vi "Load XML.vi"(8 "Error In":errorcluster, 10 "XML File":path caption="UIM XML Path", 11 "UIM In":refnum<data-value>) -> (0 "Error Out":errorcluster, 3 "UIM Out":refnum<data-value>)   [LabVIEW 2020, in "UIM.lvlib" / "UIM.lvclass"]
doc: "Overwrite the existing UIM state data with the data loaded from XML.\n\n<b>Important </b>- If the XML file specifies the <UIPList> only the plugins specified in that list will be used and loaded with the file. Make sure that the list specifies ALL the plugins used in the UIM States. Otherwise they will not be loaded. If the <UIPList> is not present in the file then the default UIPs and the UIPs from the Plugin folder will be used."
uses:
  UIM.lvclass
  <vilib>/xml/Load XML File.vi
  <vilib>/xml/Close Reference(Node).vi
  <vilib>/xml/NI_XML.lvlib
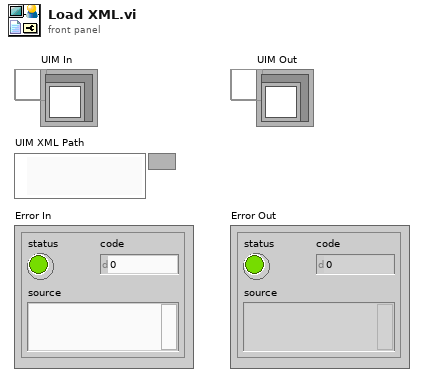
[diagram p1: front panel]
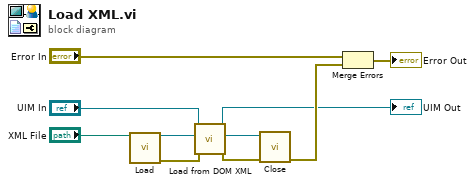
[diagram p0: block diagram]
diagram:
  n1 = call-poly <vilib>:"Load.vi"("path to XML document"="XML File") -> ("DOM document out"=w7:refnum<k20>, "error out"=w6:errorcluster)  [unwired: 12 in, 1 out]
  n2 = call "Load from DOM XML.vi"("Error In"=w6, "DOM In"=w7, "UIM In"="UIM In") -> ("Error Out"=w3:errorcluster, "DOM Out"=w4:refnum<k20>, "UIM Out"=→"UIM Out":refnum<data-value>)  [unwired: 6 in]
  n3 = call-poly <vilib>:"Close.vi"("error in (no error)"=w3, "node"=w4) -> ("error out"=w2:errorcluster)  [unwired: 7 in]
  n4 = Merge Errors("Error In", w2) -> (→"Error Out":errorcluster)
